vi "Auto Fast Pivot.vi"(10 "Pivot Speed":dbl, 11 "Heading":dbl) -> (3 "Done?":bool)   [LabVIEW 2015]
uses:
  Common Code/Drivetrain Modes.ctl
  Robot Global Data.vi
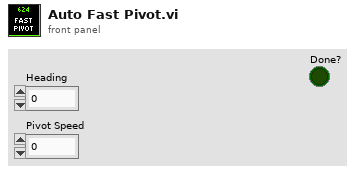
[diagram p1: front panel]
types:
  T1 = typedef "Drivetrain Modes.ctl" = enum16{"Tank", "Climb", "Manual", "Goal Vision Targeting", "PID Distance Drive", "Hybrid", "Gyro Steer"}
  T2 = typedef "Drivetrain Status Cluster.ctl" = cluster{"Modes":T1, "Y (Throttle)":dbl, "X (Steer)":dbl, "Gyro In Range?":bool, "Distance Drive Finished?":bool, "Stop Eject Lockout":bool, "Dist Drive Status":T3, "Y Target":dbl, "Heading Target":dbl, "Vision Target Aligned?":bool, "Gear":dbl, "1st Gear Time":dbl, "2nd Gear Time":dbl, "1st Gear Shifts":dbl, "2nd Gear Shifts":dbl}
  T3 = typedef "Dist Drive Status.ctl" = cluster{"Y In Range":bool, "X In Range":bool, "Gyro In Range":bool, "Y Dist":dbl, "X Dist":dbl, "Gyro":dbl}
  T4 = typedef "Drivetrain Commands.ctl" = cluster{"Y Power":dbl, "Turn Power":dbl, "1st Gear?":bool, "Modes":T1, "Heading Target":dbl, "X Max Speed":dbl, "Y Max Speed":dbl, "X Min Speed":dbl, "Y Min Speed":dbl, "Y Target":dbl, "Max Accel":dbl, "Max Velocity":dbl, "Y Power 2":dbl, "Pivot Speed":dbl}
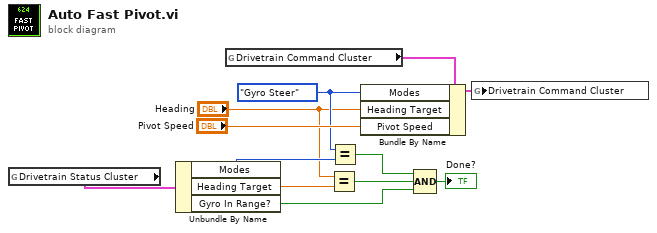
[diagram p0: block diagram]
diagram:
  w8 = Drivetrain_Modes."Gyro Steer" ("Modes")
  n1 = global read "Robot Global Data.vi" "Drivetrain Status Cluster"() -> (w12:T2)
  n2 = Unbundle By Name(w12) -> ("Modes"=w7:T1, "Heading Target"=w5:dbl, "Gyro In Range?"=w4:bool)
  n3 = global read "Robot Global Data.vi" "Drivetrain Command Cluster"() -> (w11:T4)
  n4 = Equal?(x="Heading", y=w5) -> (x = y?=w3:bool)
  n5 = Equal?(x=w8, y=w7) -> (x = y?=w2:bool)
  n6 = Bundle By Name(cluster=w11, "Modes"=w8, "Heading Target"="Heading", "Pivot Speed"="Pivot Speed") -> (w10:T4)
  n7 = Compound Arithmetic op=AND(w2, w3, w4) -> (→"Done?":bool)
  n8 = global write "Robot Global Data.vi" "Drivetrain Command Cluster"(w10) -> ()
